vi "processor piecewise.vi"(10 "application request":T1={"request id"=0, "role"=enum."none", "standard input"="", "data"="", "dictionary"=variant(cluster{"key":string, "value":string}[] []), "close after response"=FALSE}, 11 "connection":refnum<k5>) -> ()   [LabVIEW 2013]
uses:
  application request.ctl
  FCGI begin request role.ctl
  FCGI record types.ctl
  FCGI end request body.ctl
  FCGI end request protocol status.ctl
  FCGI record header.ctl
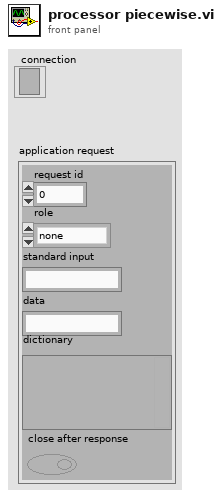
[diagram p1: front panel]
types:
  T1 = typedef "application request.ctl" = cluster{"request id":u16, "role":T2, "standard input":string, "data":string, "dictionary":variant, "close after response":bool}
  T2 = typedef "FCGI begin request role.ctl" = enum16{"none", "Responder", "Authorizer", "Filter"}
  T3 = typedef "FCGI record header.ctl" = cluster{"version":u8, "type":T4, "request id":u16, "content length":u16, "padding length":u8, "reserved":u8}
  T4 = typedef "FCGI record types.ctl" = enum8{"Error", "Begin Request", "Abort Request", "End Request", "Parameters", "Standard Input", "Standard Output", "Standard Error", "Data", "Get Values", "Get Values Result", "Unknown Type"}
  T5 = typedef "FCGI end request protocol status.ctl" = enum8{"complete", "cant mpx connection", "overloaded", "unknown role"}
  T6 = typedef "FCGI end request body.ctl" = cluster{"application status":u32, "protocol status":T5, "reserved 1":u8, "reserved 2":u8, "reserved 3":u8}
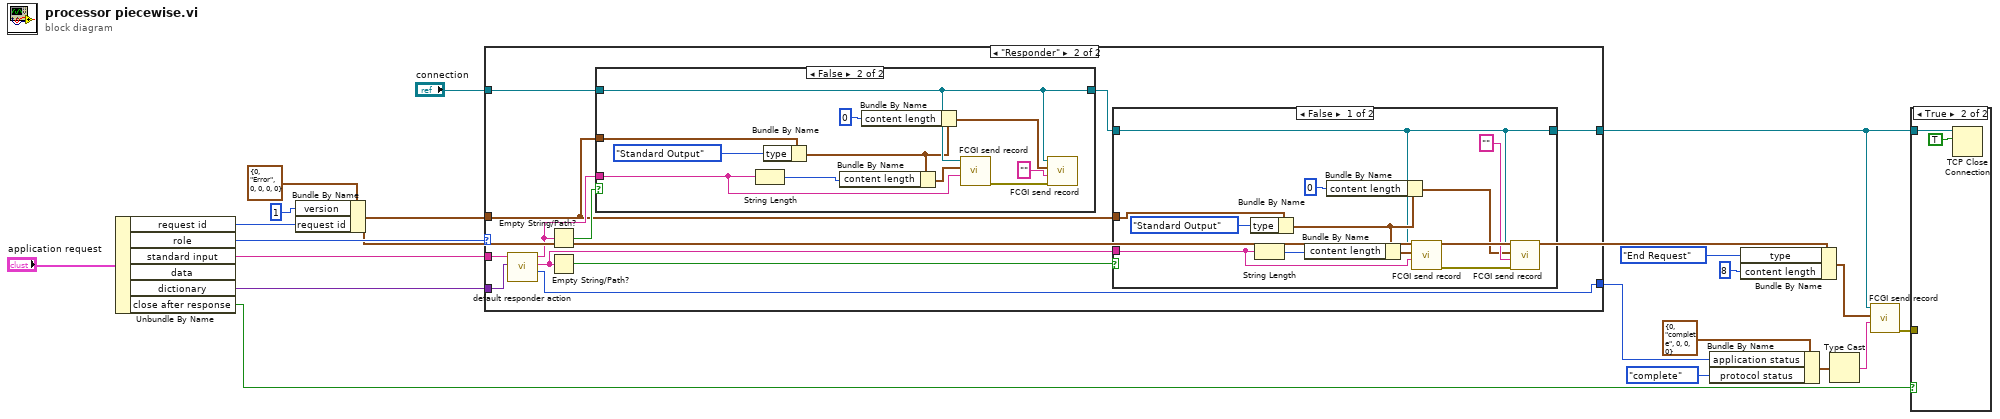
[diagram p0: block diagram]
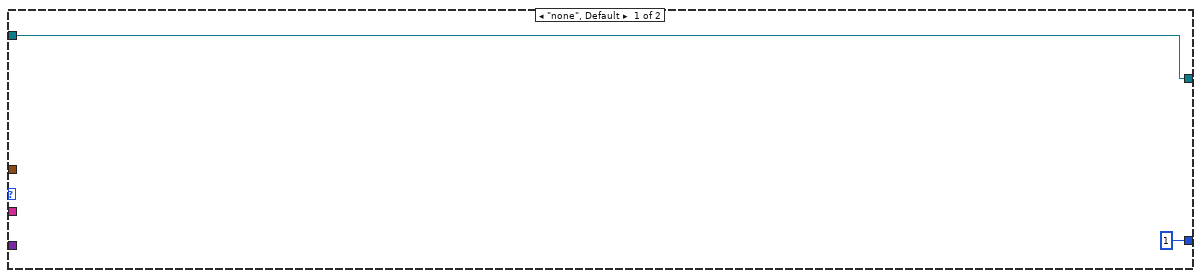
[diagram p3: hidden frame]
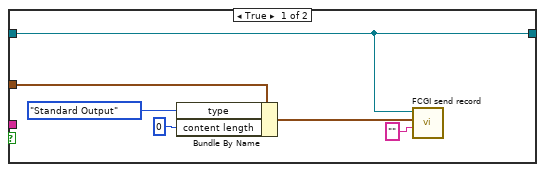
[diagram p5: hidden frame]
diagram:
  n1 = Unbundle By Name("application request") -> ("request id"=w7:u16, "role"=w19:T2, "standard input"=w16:string, "dictionary"=w15:variant, "close after response"=w17:bool)  [unwired: 1 out]
  n2 = Bundle By Name(cluster=T3 {"version"=0, "type"=enum."Error", "request id"=0, "content length"=0, "padding length"=0, "reserved"=0} ("header"), "version"=u8 1, "request id"=w7) -> (w3:T3)
  n3 = case shown="\"Responder\"" w19 {
    tunnel: "connection" -> [w22 w30]
    tunnel: [w22 w28] -> w5
    tunnel: w16 -> [_ w33]
    tunnel: w15 -> [_ w32]
    tunnel: w3 -> [_ w25]
    tunnel: [u32 1 ("code") w23] -> w1
    frame "none", Default {
    }
    frame "Responder" {
      n4 = call "default responder action.vi"("dictionary"=w32, "standard input"=w33) -> ("code"=w23:u32, "standard error"=w24:string, "standard out"=w26:string)  [unwired: 7 in]
      n5 = Empty String/Path?(string/path=w26) -> (empty?=w31:bool)
      n6 = Empty String/Path?(string/path=w24) -> (empty?=w29:bool)
      n7 = case shown="False" w31 {
        tunnel: w25 -> [w48 w60]
        tunnel: w30 -> [w47 w58]
        tunnel: [w47 w58] -> w27
        tunnel: w26 -> [_ w52]
        frame True {
          n8 = Bundle By Name(cluster=w48, "type"=FCGI_record_types."Standard Output", "content length"=u16 0) -> (w51:T3)
          n9 = call "FCGI send record.vi"("data"="", "header"=w51, "connection"=w47) -> ()  [unwired: 8 in, 1 out]
        }
        frame False {
          n10 = String Length(string=w52) -> (length=w53:i32)
          n11 = Bundle By Name(cluster=w60, "type"=FCGI_record_types."Standard Output") -> (w56:T3)
          n12 = Bundle By Name(cluster=w56, "content length"=w53) -> (w57:T3)
          n13 = Bundle By Name(cluster=w56, "content length"=u16 0) -> (w55:T3)
          n14 = call "FCGI send record.vi"("data"=w52, "header"=w57, "connection"=w58) -> ("error out"=w59:errorcluster)  [unwired: 8 in]
          n15 = call "FCGI send record.vi"("error in"=w59, "data"="", "header"=w55, "connection"=w58) -> ()  [unwired: 7 in, 1 out]
        }
      }
      n16 = case shown="False" w29 {
        tunnel: [w37 w45] -> w28
        tunnel: w27 -> [w37 w45]
        tunnel: w25 -> [w38 _]
        tunnel: w24 -> [w35 _]
        frame False {
          n17 = Bundle By Name(cluster=w38, "type"=FCGI_record_types."Standard Output") -> (w42:T3)
          n18 = String Length(string=w35) -> (length=w44:i32)
          n19 = Bundle By Name(cluster=w42, "content length"=w44) -> (w36:T3)
          n20 = Bundle By Name(cluster=w42, "content length"=u16 0) -> (w34:T3)
          n21 = call "FCGI send record.vi"("data"=w35, "header"=w36, "connection"=w37) -> ("error out"=w41:errorcluster)  [unwired: 8 in]
          n22 = call "FCGI send record.vi"("error in"=w41, "data"="", "header"=w34, "connection"=w37) -> ()  [unwired: 7 in, 1 out]
        }
        frame True {
        }
      }
    }
  }
  n23 = Bundle By Name(cluster=T6 {"application status"=0, "protocol status"=enum."complete", "reserved 1"=0, "reserved 2"=0, "reserved 3"=0} ("record header"), "application status"=w1, "protocol status"=FCGI_end_request_protocol_status."complete") -> (w11:T6)
  n24 = Bundle By Name(cluster=w3, "type"=FCGI_record_types."End Request", "content length"=u16 8) -> (w13:T3)
  n25 = Type Cast(x=w11) -> (*(type *) &x=w6:string)  [unwired: 1 in]
  n26 = call "FCGI send record.vi"("data"=w6, "header"=w13, "connection"=w5) -> ("error out"=w4:errorcluster)  [unwired: 8 in]
  n27 = case shown="True" w17 {
    tunnel: w5 -> [_ w63]
    tunnel: w4 -> [_ _]
    frame False {
    }
    frame True {
      n28 = TCP Close Connection(connection ID=w63, abort (F)=TRUE) -> ()  [unwired: 1 in, 2 out]
    }
  }
